vi "Update Data.vi"(8 "error in (no error)":errorcluster, 10 "Message Data":variant, 11 "List Seen Processes View Model In":refnum<class "Control View Model.lvclass">) -> (0 "error out":errorcluster, 3 "List Seen Processes View Model Out":refnum<class "Control View Model.lvclass">)   [LabVIEW 2020]
uses:
  Control View Model.lvclass
  Control View Model.lvclass/Control View Model.ctl
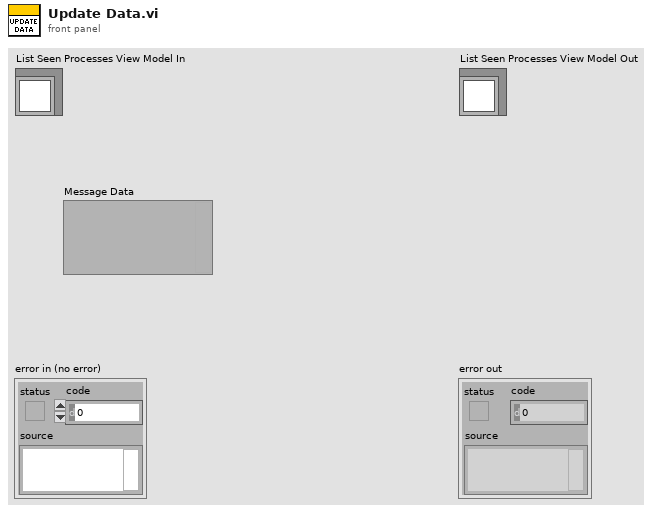
[diagram p1: front panel]
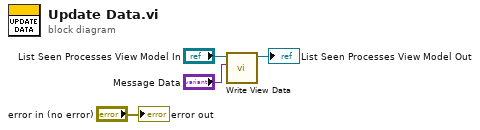
[diagram p0: block diagram]
diagram:
  n1 = call "Write View Data.vi"("View Data"="Message Data", "List Box View Model in"="List Seen Processes View Model In") -> ("List Box View Model out"=→"List Seen Processes View Model Out":refnum<class "Control View Model.lvclass">)  [unwired: 8 in, 1 out]
  "error out" <- "error in (no error)"
